vi "Battery Potentiometer.vi"(1 "Numeric":dbl) -> (0 "Low Battery\nfor potentiometer":errorcluster)   [LabVIEW 2015]
uses:
  <vilib>/ErrorRing/Error Ring.xnode
panel:
  out "Battery > 75 %":bool
  out "Battery > 50 %":bool
  out "Battery > 25%":bool
  out "Battery > 0%":bool
  out "timed out?\nBattery potentiometer":bool
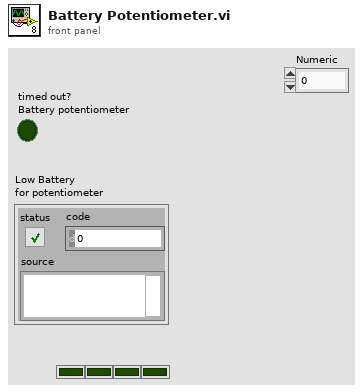
[diagram p1: front panel]
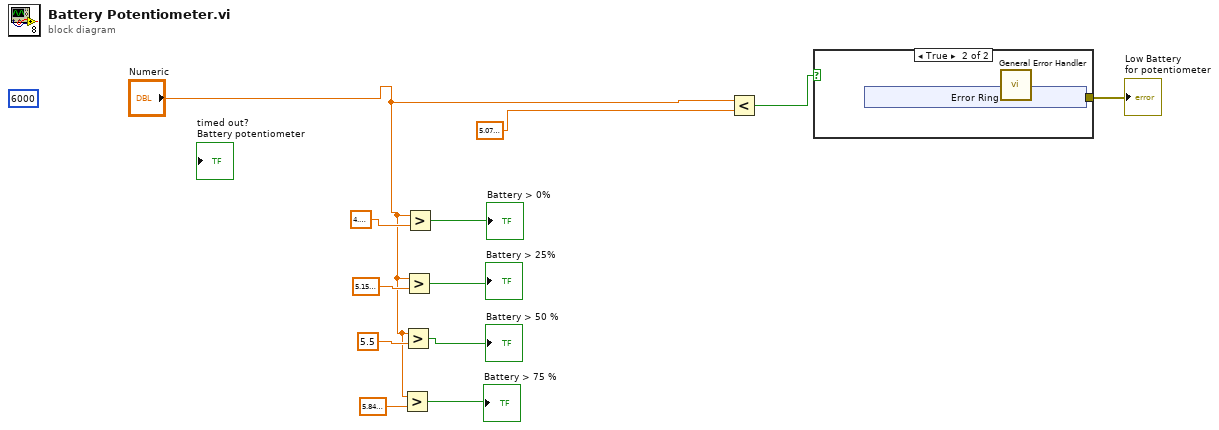
[diagram p0: block diagram]
diagram:
  (unwired) 6000 ("ms timeout (0)")
  n1 = Greater?(x="Numeric", y=sgl 5.85) -> (0:→"Battery > 75 %":bool)
  n2 = Greater?(x="Numeric", y=sgl 5.5) -> (0:→"Battery > 50 %":bool)
  n3 = Greater?(x="Numeric", y=sgl 5.15) -> (0:→"Battery > 25%":bool)
  n4 = Greater?(x="Numeric", y=sgl 4.8) -> (0:→"Battery > 0%":bool)
  n5 = Less?(x="Numeric", y=sgl 5.08) -> (x < y?=w10:bool)
  n6 = case shown="True" w10 {
    tunnel: [_ w14] -> w12
    frame False {
    }
    frame True {
      n7 = xnode "Error Ring"() -> ("error out"=w13:errorcluster)
      n8 = call <vilib>:"General Error Handler.vi"("error in (no error)"=w13) -> ("error out"=w14:errorcluster)  [unwired: 10 in, 4 out]
    }
  }
  "Low Battery\nfor potentiometer" <- w12
